vi "User Console View.vi"(8 "error in (no error)":errorcluster, 11 "View Model":T3) -> (0 "error out":errorcluster)   [LabVIEW 2017]
doc: "The interface where a user enters information and responds to system prompts.\n[Covers: UI2]"
uses:
  View Model/Controls/View Model.ctl
  View Model/Controls/Shared Model.ctl
  Error Handler/Controls/Error Model.ctl
  Error Handler/Controls/Error Data.ctl
  Error Handler/Controls/Error Type.ctl
  Error Handler/Controls/Error Source.ctl
  Configuration/Controls/Config Model.ctl
  Configuration/Controls/Config CMD.ctl
  Configuration/Controls/Config Command.ctl
  Controller/Controls/Controller Model.ctl
  Controller/Controls/Controller Overhead.ctl
  Controller/Controls/Controller Transaction.ctl
  Controller/Controls/Controller State.ctl
  Configuration/Controls/Config Data Record.ctl
  Controls/User Console - Keypad.ctl
  Controls/User Console - Transactions.ctl
  Controls/User Console - References.ctl
panel:
  in  "Transactions":T1
  in  "Card Reader":bool
  in  "Keypad":T2
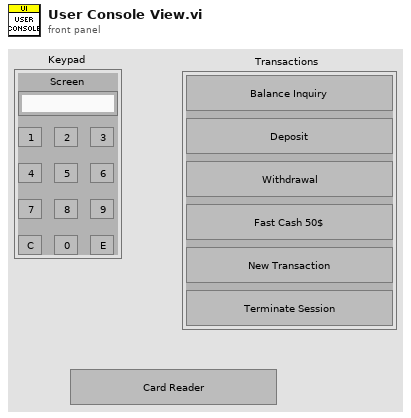
[diagram p1: front panel]
types:
  T1 = typedef "User Console - Transactions.ctl" = cluster{"Balance Inquiry":bool, "Deposit":bool, "Withdrawal":bool, "Fast Cash":bool, "New Transaction":bool, "Terminate Session":bool}
  T2 = typedef "User Console - Keypad.ctl" = cluster{"Screen":string, "1":bool, "2":bool, "3":bool, "4":bool, "5":bool, "6":bool, "7":bool, "8":bool, "9":bool, "C":bool, "0":bool, "E":bool}
  T3 = typedef "View Model.ctl" = cluster{"Shared Model":T4, "Error Model":T5, "Config Model":T6, "Controller Model":T7}
  T4 = typedef "Shared Model.ctl" = cluster{"Stop":refnum<user-event>, "Stop DVR":refnum<data-value>}
  T5 = typedef "Error Model.ctl" = cluster{"Error":refnum<user-event>}
  T6 = typedef "Config Model.ctl" = cluster{"Config CMD":refnum<user-event>}
  T7 = typedef "Controller Model.ctl" = cluster{"Deposit Received":refnum<user-event>, "Funds Dispensed":refnum<user-event>, "Overhead DVR":refnum<data-value>, "Entered Num":refnum<user-event>, "Card Read":refnum<user-event>, "Transaction":refnum<user-event>}
  T8 = typedef "User Console - References.ctl" = cluster{"Transactions":refnum<vi>, "Card Reader":refnum<vi>, "Keypad":refnum<vi>}
  T9 = enum8{"Enabled", "Disabled", "Disabled and Grayed Out"}
  T10 = typedef "Controller State.ctl" = enum16{"Idle", "Initial", "Login", "Balance Inquiry", "Deposit", "Withdrawal", "Fast Cash", "Terminate"}
  T11 = typedef "Controller Transaction.ctl" = enum16{"Balance Inquiry", "Deposit", "Withdrawal", "Fast Cash", "New Transaction", "Terminate Session"}
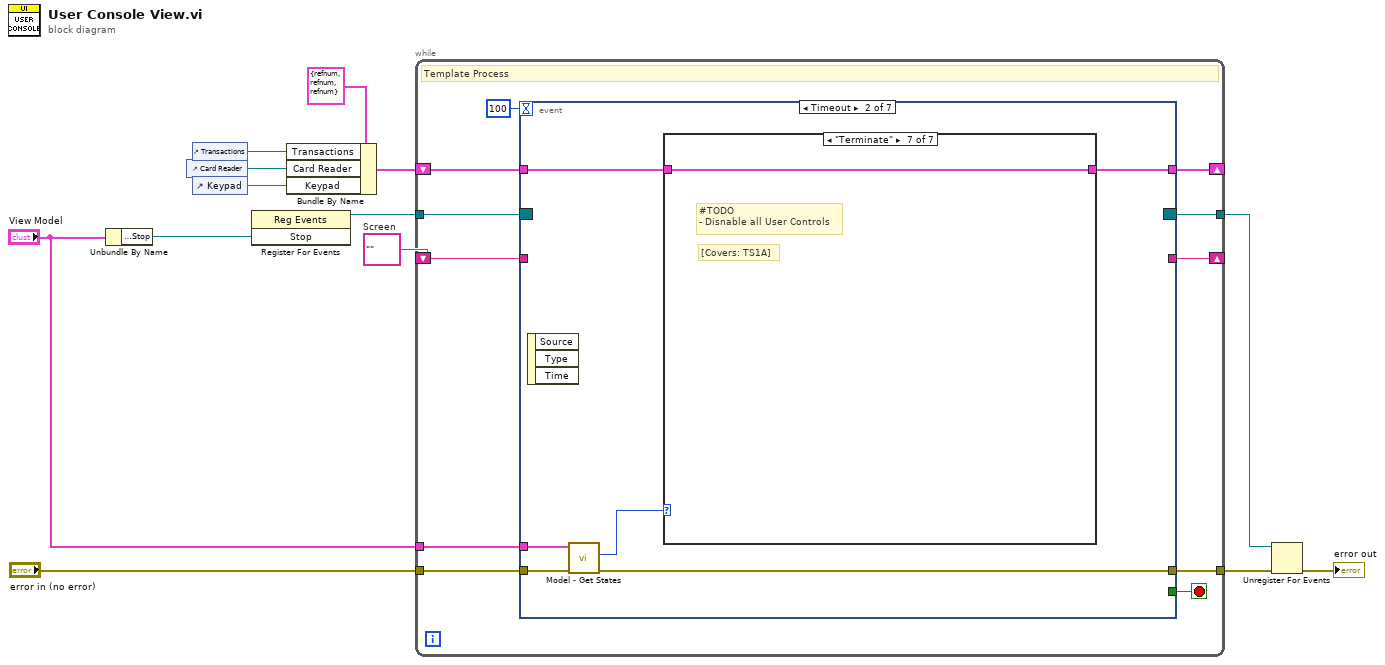
[diagram p0: block diagram]
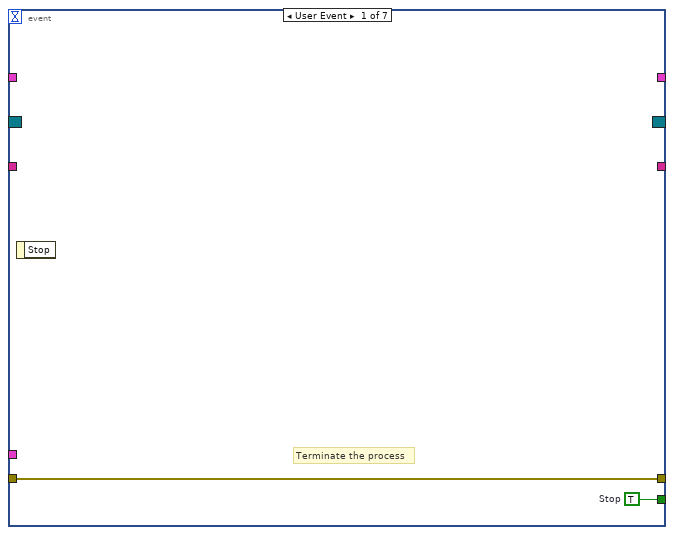
[diagram p2: hidden frame]
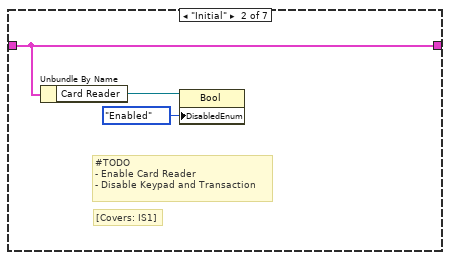
[diagram p4: hidden frame]
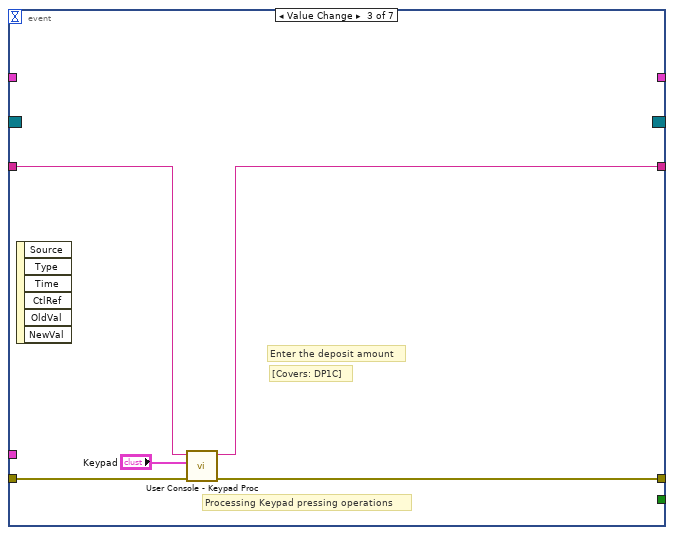
[diagram p9: hidden frame]
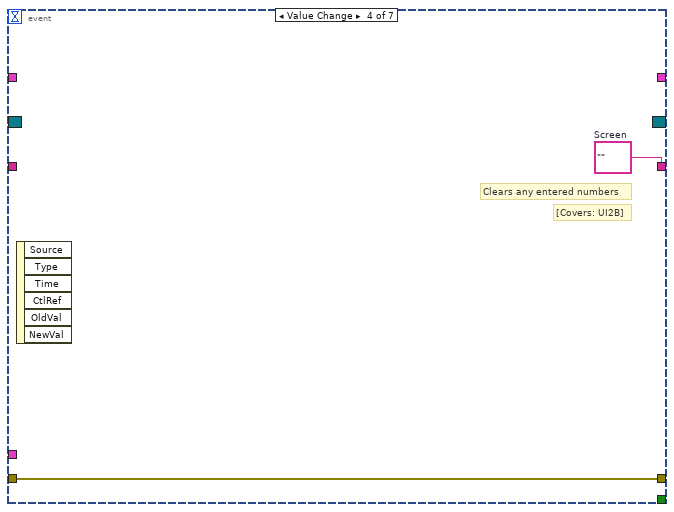
[diagram p10: hidden frame]
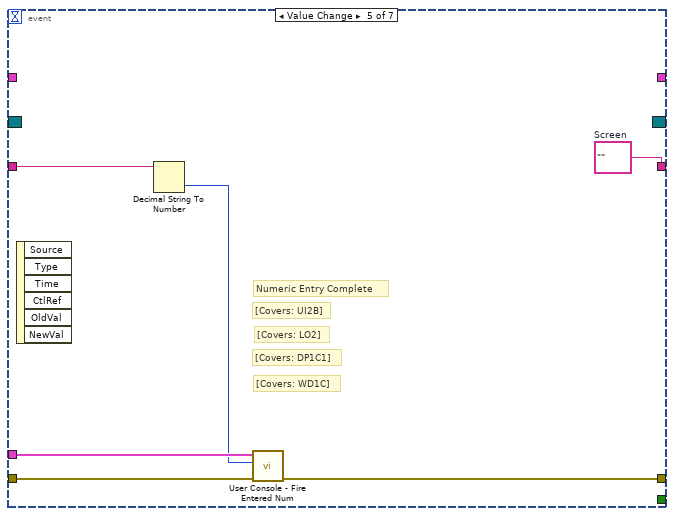
[diagram p11: hidden frame]
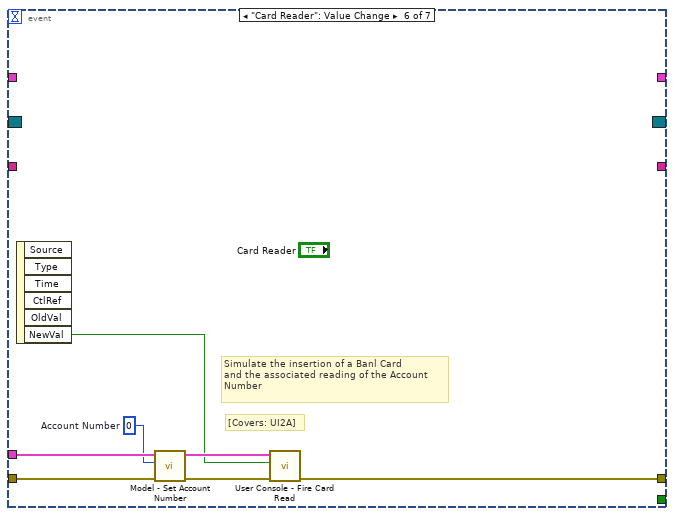
[diagram p12: hidden frame]
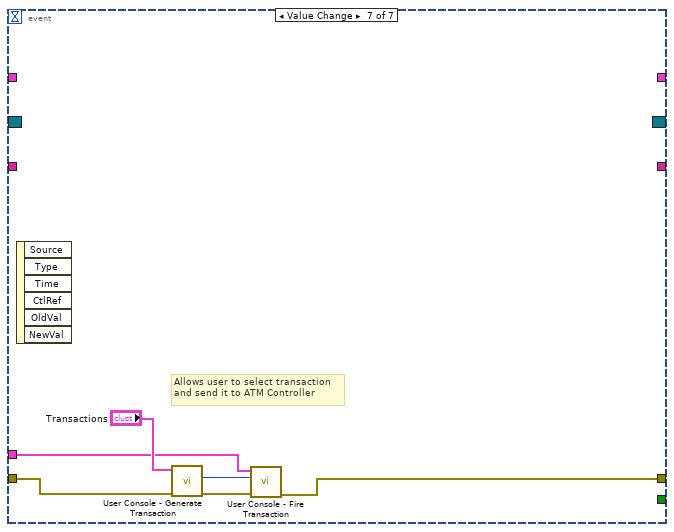
[diagram p13: hidden frame]
diagram:
  w6 = ""  # Screen
  n1 = Unbundle By Name("View Model") -> ("Shared Model.Stop"=w13:refnum<user-event>)
  n2 = control-ref of="Card Reader"() -> (w1:refnum<vi>)
  n3 = control-ref of="Transactions"() -> (w3:refnum<vi>)
  n4 = control-ref of="Keypad"() -> (w2:refnum<vi>)
  n5 = register-events(w13) -> (reference out=w12:refnum<event-registration>)  [unwired: 2 in, 1 out]
  n6 = Bundle By Name(cluster=T8 {"Transactions"=refnum, "Card Reader"=refnum, "Keypad"=refnum} ("References"), "Transactions"=w3, "Card Reader"=w1, "Keypad"=w2) -> (w4:T8)
  n7 = while {
    tunnel: w12 -> [w24]
    tunnel: [w23] -> w11
    tunnel: "error in (no error)" -> [w22]
    tunnel: [w21] -> w8
    tunnel: "View Model" -> [w17]
    shift-right: [w18] -> _
    shift-left: w6 -> [w19]
    shift-right: [w14] -> _
    shift-left: w4 -> [w16]
    stop <- w20 stop-if-true
    # "Template Process"
    n8 = event shown="[1] Timeout" {
      selector: w24 -> [_ _ _ _ _ _ _]
      dyn-events: [_ _ _ _ _ _ _] -> w23
      timeout: 100 -> [_ _ _ _ _ _ _]
      tunnel: w22 -> [w26 w32 w46 w48 w52 w61 w67]
      tunnel: [w26 w30 w45 w48 w51 w55 w62] -> w21
      tunnel: [w25 _ _ _ _ _ _] -> w20
      tunnel: w19 -> [_ _ w43 _ w53 _ _]
      tunnel: [_ _ w42 w47 w54 _ _] -> w18
      tunnel: w17 -> [_ w31 _ _ w50 w60 w64]
      tunnel: w16 -> [_ w28 _ _ _ _ _]
      tunnel: [_ w27 _ _ _ _ _] -> w14
      event User Event {
        w25 = TRUE  # Stop
        # "Terminate the process"
        n9 = event-data() -> ()  [unwired: 1 in, 1 out]
      }
      event Timeout {
        n10 = event-data() -> ()  [unwired: 1 in, 3 out]
        n11 = call "Model - Get States.vi"("error in (no error)"=w32, "View Model"=w31) -> ("error out"=w30:errorcluster, "Current State"=w29:T10)  [unwired: 6 in, 2 out]
        n12 = case shown="\"Terminate\"" w29 {
          tunnel: w28 -> [w33 w34 w37 w38 w39 w40 w41]
          tunnel: [w33 w34 w37 w38 w39 w40 w41] -> w27
          frame "Idle", Default {
            # "[Covers: ID1A]"
            # "#TODO\n- Disable Card Reader and set it ON\n- Disable Keypad\n- Enable all Transaction\n(use \"Initial\" state as example)"
          }
          frame "Initial" {
            # "[Covers: IS1]"
            # "#TODO\n- Enable Card Reader\n- Disable Keypad and Transaction"
            n13 = Unbundle By Name(w34) -> ("Card Reader"=w36:refnum<vi>)
            n14 = property class="Bool"(reference=w36, "DisabledEnum"=T9."Enabled" ("Disabled")) -> ()  [unwired: 1 in, 2 out]
          }
          frame "Login" {
            # "[Covers: LO1A]"
            # "#TODO\n- Disable Card Reader and remain it ON\n- Enable Keypad\n- Disnable all Transaction except Terminate Session \n(use \"Initial\" state as example)"
          }
          frame "Deposit" {
            # "[Covers: DP1A]"
            # "#TODO\n- Enable Keypad\n- Disnable all Transaction except Terminate Session\nAND New Transaction \n(use \"Initial\" state as example)"
          }
          frame "Withdrawal" {
            # "[Covers: WD1A]"
            # "#TODO\n- Enable Keypad\n- Disnable all Transaction except Terminate Session\nAND New Transaction \n(use \"Initial\" state as example)"
          }
          frame "Fast Cash" {
            # "[Covers: FC1A]"
            # "#TODO\n- Disnable all Transaction except Terminate Session\nAND New Transaction \n(use \"Initial\" state as example)"
          }
          frame "Terminate" {
            # "[Covers: TS1A]"
            # "#TODO\n- Disnable all User Controls"
          }
        }
      }
      event Value Change {
        # "[Covers: DP1C]"
        # "Enter the deposit amount"
        # "Processing Keypad pressing operations"
        n15 = event-data() -> ()  [unwired: 1 in, 6 out]
        n16 = call "User Console - Keypad Proc.vi"("error in (no error)"=w46, "Keypad"="Keypad", "Screen"=w43) -> ("error out"=w45:errorcluster, "Screen"=w42:string)  [unwired: 7 in]
      }
      event Value Change {
        w47 = ""  # Screen
        # "[Covers: UI2B]"
        # "Clears any entered numbers"
        n17 = event-data() -> ()  [unwired: 1 in, 6 out]
      }
      event Value Change {
        w54 = ""  # Screen
        # "[Covers: WD1C]"
        # "[Covers: DP1C1]"
        # "[Covers: LO2]"
        # "Numeric Entry Complete"
        # "[Covers: UI2B]"
        n18 = event-data() -> ()  [unwired: 1 in, 6 out]
        n19 = Decimal String To Number(string=w53) -> (number=w49:i32)  [unwired: 2 in, 1 out]
        n20 = call "User Console - Fire Entered Num.vi"("error in (no error)"=w52, "Entered Num"=w49, "View Model"=w50) -> ("error out"=w51:errorcluster)  [unwired: 7 in, 1 out]
      }
      event "Card Reader": Value Change {
        w56 = u32 0  # Account Number
        # "[Covers: UI2A]"
        # "Simulate the insertion of a Banl Card\nand the associated reading of the Account\nNumber"
        n21 = event-data() -> ("NewVal"=w57:bool)  [unwired: 1 in, 5 out]
        n22 = call "Model - Set Account Number.vi"("error in (no error)"=w61, "Account Number"=w56, "View Model"=w60) -> ("error out"=w59:errorcluster, "View Model"=w58:T3)  [unwired: 7 in]
        n23 = call "User Console - Fire Card Read.vi"("error in (no error)"=w59, "Card Read"=w57, "View Model"=w58) -> ("error out"=w55:errorcluster)  [unwired: 7 in, 1 out]
      }
      event Value Change {
        # "Allows user to select transaction\nand send it to ATM Controller"
        n24 = event-data() -> ()  [unwired: 1 in, 6 out]
        n25 = call "User Console - Generate Transaction.vi"("error in (no error)"=w67, "Transactions"="Transactions") -> ("error out"=w65:errorcluster, "Transaction"=w63:T11)  [unwired: 8 in]
        n26 = call "User Console - Fire Transaction.vi"("error in (no error)"=w65, "Transaction"=w63, "View Model"=w64) -> ("error out"=w62:errorcluster)  [unwired: 7 in, 1 out]
      }
    }
  }
  n27 = Unregister For Events(event registration refnum=w11, error in=w8) -> (error out=→"error out":errorcluster)
